vi "ma_SML RT Zoom FFT (real input).vi"(6 "reset?":bool, 7 "export time data?":bool, 8 "error in (no error)":errorcluster, 9 "zoom FFT settings":T2={"zoom settings"={"center frequency"=-inf, "zoom"=1, "trim"=1.0}, "FFT settings"={"window"=1, "window size"=-1, "FFT size"=1024, "%overlap"=0.0}} {"FFT settings"."%overlap" min=0.0 max=100.0 format="%.2f"; "FFT settings"."window" items=["Rectangle"=0, "Hanning"=1, "Hamming"=2, "Blackman-Harris"=3, "Exact Blackman"=4, "Blackman"=5, "Flat Top"=6, "4 Term B-Harris "=7, "7 Term B-Harris"=8, "Low Sidelobe"=9, "Blackman Nuttall"=11, "Triangle"=30, "Bartlett-Hanning"=31, "Bohman"=32, "Parzen"=33, "Welch"=34, "Kaiser"=60, "Dolph-Chebyshev"=61, "Gaussian"=62]; "zoom settings"."trim" min=1.0 format="%.2f"; "zoom settings"."center frequency" format="%.2f"; "zoom settings"."zoom" min=1}, 10 "fs":dbl=1024.0 format="%.2f", 11 "x":dbl[](array[numeric]) format="%.2f") -> (0 "error out":errorcluster, 1 "spectrum ready":bool, 2 "spectral info":T3 {"window" items=["Rectangle"=0, "Hanning"=1, "Hamming"=2, "Blackman-Harris"=3, "Exact Blackman"=4, "Blackman"=5, "Flat Top"=6, "4 Term B-Harris "=7, "7 Term B-Harris"=8, "Low Sidelobe"=9, "Blackman Nuttall"=11, "Triangle"=30, "Bartlett-Hanning"=31, "Bohman"=32, "Parzen"=33, "Welch"=34, "Kaiser"=60, "Dolph-Chebyshev"=61, "Gaussian"=62]}, 3 "FFT spectrum":T4 {"spectrum" format="%.2f"; "df" format="%.2f"; "f0" format="%.2f"}, 5 "time data":T1 {"data" format="%.2f"; "dt" format="%.2f"; "t0" format="%.2f"})   [LabVIEW 2020, in "NI_MAPro.lvlib"]
uses:
  NI_MAPro.lvlib
  ma_sml_Spectrum Cluster (complex).ctl
  ma_sml_Spectral Info.ctl
  ma_sml_RT Zoom FFT Settings.ctl
  NI_AALPro.lvlib
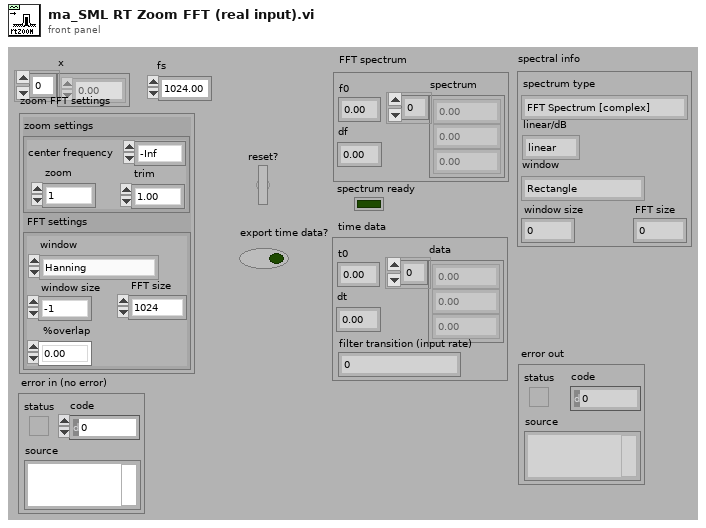
[diagram p1: front panel]
types:
  T1 = cluster{"t0":dbl, "dt":dbl, "data":cdb[], "filter transition (input rate)":i32}
  T2 = typedef "NI_MAPro.lvlib/ma_sml_RT Zoom FFT Settings.ctl" = cluster{"zoom settings":cluster{"center frequency":dbl, "zoom":i32, "trim":dbl}, "FFT settings":cluster{"window":u16, "window size":i32, "FFT size":i32, "%overlap":dbl}}
  T3 = typedef "NI_MAPro.lvlib/ma_sml_Spectral Info.ctl" = cluster{"spectrum type":enum16{"FFT Spectrum [complex]", "Amplitude [Magnitude]", "Power [Magnitude^2]", "Cross Spectrum [complex]", "Frequency Response [Complex]"}, "linear/dB":enum16{"linear", "dB"}, "window":u16, "window size":i32, "FFT size":i32}
  T4 = typedef "NI_MAPro.lvlib/ma_sml_Spectrum Cluster (complex).ctl" = cluster{"f0":dbl, "df":dbl, "spectrum":cdb[]}
  T5 = cluster{"center frequency":dbl, "zoom":i32, "trim":dbl}
  T6 = cluster{"window":u16, "window size":i32, "FFT size":i32, "%overlap":dbl}
  T7 = cluster{"zoom":i32, "stop band attenuation":enum16{"84 dB", "96 dB", "120 dB"}, "alias protect in final transition":bool, "oversampling ratio":dbl}
  T8 = cluster{"x":dbl, "dt":dbl, "Time data":cdb[], "filter transition length":i32}
  T9 = cluster{"x":dbl, "dt":dbl, "time data":cdb[], "filter transition length":i32}
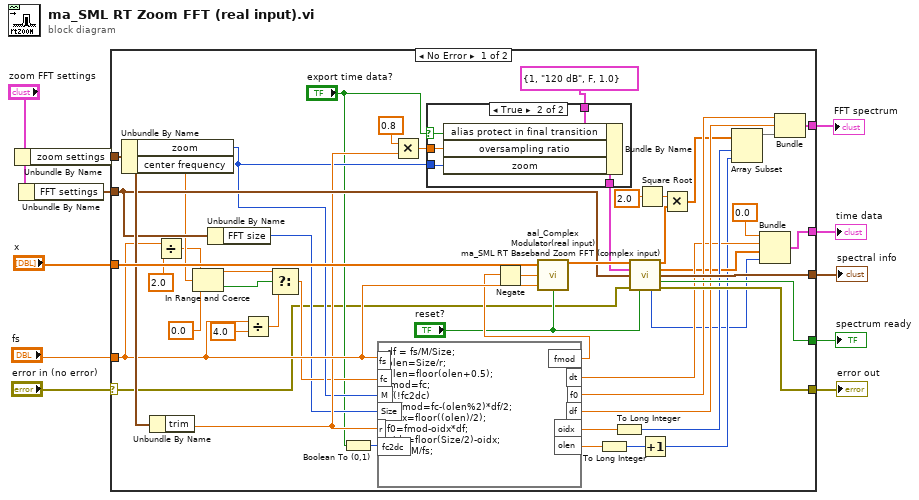
[diagram p0: block diagram]
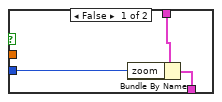
[diagram p2: hidden frame]
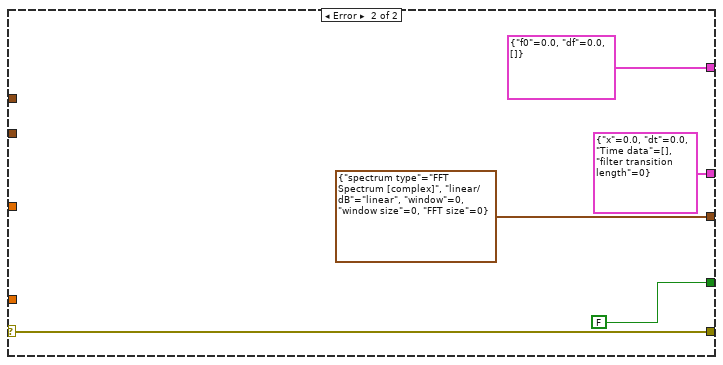
[diagram p3: hidden frame]
diagram:
  n1 = Unbundle By Name("zoom FFT settings") -> ("zoom settings"=w4:T5)
  n2 = Unbundle By Name("zoom FFT settings") -> ("FFT settings"=w3:T6)
  n3 = case shown="No Error" "error in (no error)" {
    selector: "error in (no error)" -> [w12 w69]
    tunnel: [w27 T8 {"x"=0.0, "dt"=0.0, "Time data"=[], "filter transition length"=0}] -> w2
    tunnel: [w59 FALSE ("SpectrumReady")] -> w11
    tunnel: w4 -> [w50 _]
    tunnel: "x" -> [w58 _]
    tunnel: "fs" -> [w36 _]
    tunnel: [w43 cluster{"f0":dbl, "df":dbl, cdb[]} {"f0"=0.0, "df"=0.0, []}] -> w9
    tunnel: [w57 T3 {"spectrum type"=enum."FFT Spectrum [complex]", "linear/dB"=enum."linear", "window"=0, "window size"=0, "FFT size"=0} ("spectral info")] -> w7
    tunnel: [w56 w69] -> w8
    tunnel: w3 -> [w41 _]
    frame No Error {
      n4 = Unbundle By Name(w50) -> ("zoom"=w19:i32, "center frequency"=w39:dbl)
      n5 = Unbundle By Name(w50) -> ("trim"=w24:dbl)
      n6 = Divide(x=w36, y=2.0) -> (x/y=w34:dbl)
      n7 = In Range and Coerce(upper limit=w34, x=w39, lower limit=0.0) -> (coerced(x)=w33:dbl, In Range?=w38:bool)
      n8 = Unbundle By Name(w41) -> ("FFT size"=w16:i32)
      n9 = Divide(x=w36, y=4.0) -> (x/y=w51:dbl)
      n10 = Select(t=w33, s=w38, f=w51) -> (s? t:f=w18:dbl)
      n11 = Boolean To (0,1)(Boolean="export time data?") -> (0, 1=w14:i16)
      n12 = formula code="df = fs/M/Size;\nolen=Size/r;\nolen=floor(olen+0.5);\nfmod=fc;\nif(!fc2dc)\n    fmod=fc-(olen%2)*df/2;\noidx=floor((olen)/2);\nf0=fmod-oidx*df;\noidx=floor(Size/2)-oidx;\ndt = M/fs;"("fc"=w18, "M"=w19, "Size"=w16, "fs"=w36, "r"=w24, "fc2dc"=w14) -> ("f0"=w48:dbl, "df"=w49:dbl, "oidx"=w47:dbl, "olen"=w46:dbl, "dt"=w30:dbl, "fmod"=w17:dbl)
      n13 = Multiply(x=0.8, y=w24) -> (x*y=w23:dbl)
      n14 = case shown="True" "export time data?" {
        selector: "export time data?" -> [_ w65]
        tunnel: T7 {"zoom"=1, "stop band attenuation"=enum."120 dB", "alias protect in final transition"=FALSE, "oversampling ratio"=1.0} ("zoom settings") -> [w62 w67]
        tunnel: [w61 w66] -> w31
        tunnel: w19 -> [w60 w63]
        tunnel: w23 -> [_ w64]
        frame False {
          n15 = Bundle By Name(cluster=w62, "zoom"=w60) -> (w61:T7)
        }
        frame True {
          n16 = Bundle By Name(cluster=w67, "alias protect in final transition"=w65, "oversampling ratio"=w64, "zoom"=w63) -> (w66:T7)
        }
      }
      n17 = Negate(x=w17) -> (-x=w42:dbl)
      n18 = call "aal_Complex Modulator(real input).vi"("reset ?"="reset?", "fs"=w36, "frequency"=w42, "x"=w58) -> ("y"=w53:cdb[])
      n19 = To Long Integer(number=w46) -> (32bit integer=w44:i32)
      n20 = To Long Integer(number=w47) -> (32bit integer=w45:i32)
      n21 = call "ma_SML RT Baseband Zoom FFT (complex input).vi"("x [V]"=w53, "zoom settings"=w31, "FFT settings"=w41, "error in (no error)"=w12, "reset?"="reset?") -> ("FFT{X} [Vrms]"=w54:cdb[], "time data"=w29:cdb[], "spectral info"=w57:T3, "spectrum ready?"=w59:bool, "filter transition length"=w25:i32, "error out"=w56:errorcluster)  [unwired: 5 in]
      n22 = Square Root(x=2.0) -> (sqrt(x)=w52:dbl)
      n23 = Increment(x=w44) -> (x+1=w26:i32)
      n24 = Multiply(x=w52, y=w54) -> (x*y=w21:cdb[])
      n25 = Array Subset(array=w21, index=w45, length=w26) -> (w20:cdb[])
      n26 = Bundle("x"=0.0, "dt"=w30, "time data"=w29, "filter transition length"=w25) -> (w27:T9)  [unwired: 1 out]
      n27 = Bundle("f0"=w48, "df"=w49, w20) -> (w43:cluster{"f0":dbl, "df":dbl, cdb[]})  [unwired: 1 out]
    }
    frame Error {
    }
  }
  "spectrum ready" <- w11
  "FFT spectrum" <- w9
  "error out" <- w8
  "spectral info" <- w7
  "time data" <- w2
